vi "Untitled 10.vi"() -> ()   [LabVIEW 2012]
panel:
  out "Output":string
  out "error out":errorcluster
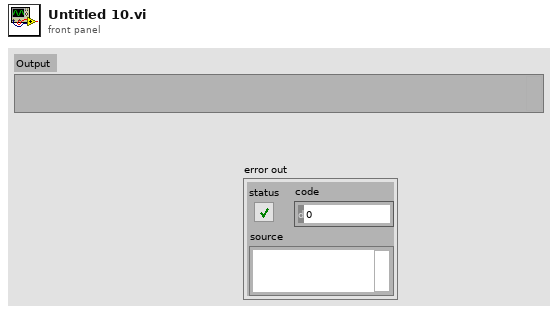
[diagram p1: front panel]
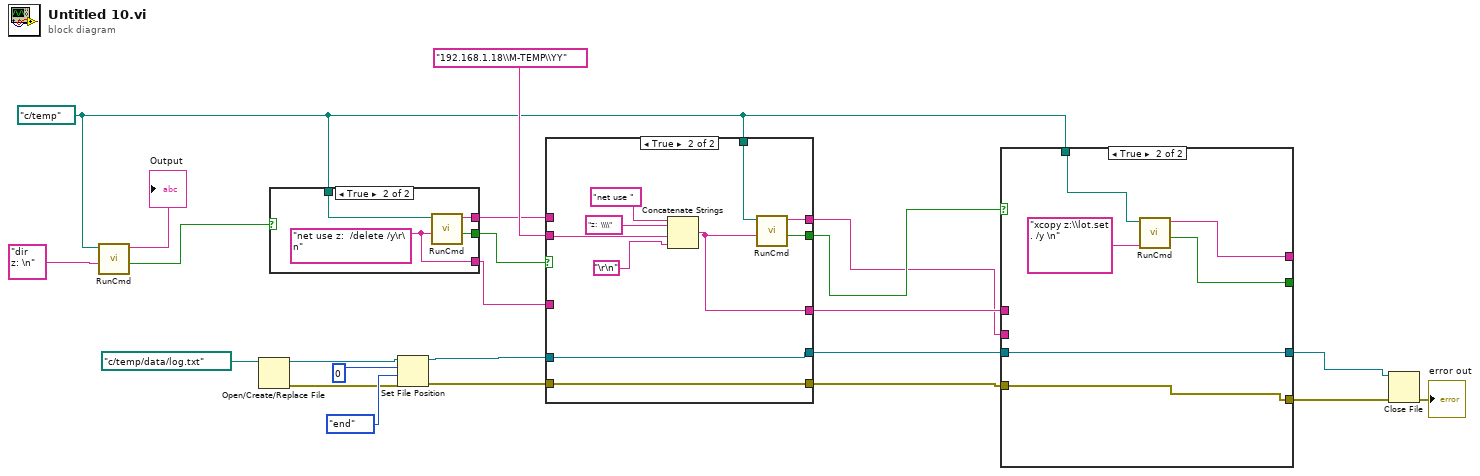
[diagram p0: block diagram]
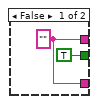
[diagram p3: hidden frame]
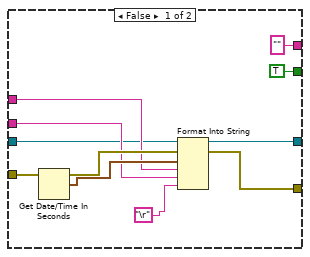
[diagram p4: hidden frame]
diagram:
  w9 = path "c:/temp" ("working directory")
  n1 = call "RunCmd.vi"("Cmd String"="dir z: \n", "working directory"=w9) -> ("OK"=w8:bool, "Output"=→"Output":string)  [unwired: 8 in]
  n2 = Open/Create/Replace File(file path (use dialog)=path "c:/temp/data/log.txt" ("input file")) -> (refnum out=w19:refnum<file>, error out=w18:errorcluster)  [unwired: 5 in, 1 out]
  n3 = case shown="True" w8 {
    tunnel: w9 -> [_ w29]
    tunnel: [TRUE ("OK") w28] -> w7
    tunnel: [w24 w27] -> w3
    tunnel: [w24 w26] -> w4
    frame False {
      w24 = "" ("Output")
    }
    frame True {
      w26 = "net use z:  /delete /y\r\n" ("Cmd String")
      n4 = call "RunCmd.vi"("Cmd String"=w26, "working directory"=w29) -> ("OK"=w28:bool, "Output"=w27:string)  [unwired: 8 in]
    }
  }
  n5 = Set File Position(offset (in bytes) (0)=i64 0, refnum=w19, from (0:start)=enum16{"start", "end", "current"}."end", error in=w18) -> (refnum out=w6:refnum<file>, error out=w5:errorcluster)
  n6 = case shown="True" w7 {
    selector: w7 -> [w30 _]
    tunnel: "192.168.1.18\\M-TEMP\\YY" -> [_ w44]
    tunnel: [w32 w40] -> w12
    tunnel: [w30 w39] -> w11
    tunnel: [w31 w38] -> w10
    tunnel: w9 -> [_ w37]
    tunnel: w6 -> [w33 w36]
    tunnel: w5 -> [w34 w35]
    tunnel: w4 -> [w32 _]
    tunnel: w3 -> [w31 _]
    tunnel: [w33 w36] -> w2
    tunnel: [w34 w35] -> w1
    frame False {
    }
    frame True {
      n7 = Concatenate Strings("net use " ("string"), "z:  \\\\" ("string"), w44, "\r\n") -> (w40:string)
      n8 = call "RunCmd.vi"("Cmd String"=w40, "working directory"=w37) -> ("OK"=w39:bool, "Output"=w38:string)  [unwired: 8 in]
    }
  }
  n9 = case shown="True" w11 {
    tunnel: [TRUE ("OK") w58] -> _
    tunnel: ["" ("Output") w57] -> _
    tunnel: w9 -> [_ w60]
    tunnel: [w54 w56] -> w15
    tunnel: [w53 w55] -> w14
    tunnel: w1 -> [w52 w55]
    tunnel: w12 -> [w50 _]
    tunnel: w10 -> [w49 _]
    tunnel: w2 -> [w47 w56]
    frame False {
      n10 = Get Date/Time In Seconds() -> (seconds since 1Jan1904=w51:timestamp)
      n11 = Format Into String(initial string=w47, error in=w52, w51, w50, w49, "\r") -> (resulting string=w54:refnum<file>, error out=w53:errorcluster)  [unwired: 1 in]
    }
    frame True {
      n12 = call "RunCmd.vi"("Cmd String"="xcopy z:\\lot.set . /y \n" ("standard input"), "working directory"=w60) -> ("OK"=w58:bool, "Output"=w57:string)  [unwired: 8 in]
    }
  }
  n13 = Close File(refnum=w15, error in=w14) -> (error out=→"error out":errorcluster)  [unwired: 1 out]
